vi "ge_CalibrateDynamic.vi"(5 "Chassis Name":string="cDAQ1", 7 "Selected Rows":i32[](array[numeric])=[0, 1, 2, 3], 8 "error in":errorcluster, 10 "ge_DAQManDefinitions":T1, 11 "ItemNames":string[][](array[string])=[["Mod1/ai0", "NI 9234", "", "", "F", "1000.00", "V", "2 mA", "5 V", "F", "1.000000", "1", "EU", "RMS"], ["Mod1/ai1", "NI 9234", "", "", "F", "1000.00", "V", "2 mA", "5 V", "F", "1.000000", "1", "EU", "RMS"], ["Mod1/ai2", "NI 9234", "", "", "F", "1000.00", "V", "2 mA", "5 V", "F", "1.000000", "1", "EU", "RMS"], ["Mod1/ai3", "NI 9234", "", "", "F", "1000.00", "V", "2 mA", "5 V", "F", "1.000000", "1", "EU", "RMS"]]) -> (0 "error out":errorcluster, 2 "Cell Contents":T2[](array[typedef]))   [LabVIEW 2018]
uses:
  Custom Ctls Table/ge_CellContents.ctl
  <vilib>/Utility/miscctls.llb/LVPoint32TypeDef.ctl
  Common/Controls/DAQMan Definitions.ctl
  ge_GrphTblCmnds.ctl
  Custom Ctrls/ge_MeasType.ctl
  Classes/Measurements/Class Dynamic/Dynamic.lvclass
  <vilib>/addons/_NISVFA/_Shared subVIs/Controls/svc_Window.ctl
  <vilib>/DAQmx/read.llb/DAQmx Read (Analog 1D Wfm NChan NSamp).vi
  <vilib>/addons/_NISVFA/_Spectrum Processing/SVFA Spectrum Peak Search (1 Ch).vi
  <vilib>/addons/_NISVFA/_Spectrum Processing/subVIs/svfa_Spectrum Peak Search.vi
  <vilib>/addons/_NISVFA/_Shared subVIs/Common/svc_Spectrum Units.vi
  <vilib>/addons/_NISVFA/_Spectrum Processing/subVIs/svfa_Peak Rough Search Indices.vi
  <vilib>/DAQmx/configure/timing.llb/DAQmx Timing (Sample Clock).vi
  <vilib>/DAQmx/miscellaneous.llb/DAQmx Fill In Error Info.vi
  <vilib>/addons/_NISVFA/_Baseband FFT/SVFA Power Spectrum (1 Ch).vi
  <vilib>/addons/_NISVFA/_Spectrum Processing/subVIs/svfa_Three Finger Peak Search.vi
  <vilib>/addons/_NISVFA/_Shared subVIs/Common/svc_Format Value (DBL).vi
  <vilib>/addons/_NISVFA/_Shared subVIs/Common/svc_Engineering Units to Unit Label.vi
  <vilib>/addons/_NISVFA/_Shared subVIs/Common/svc_Unit Label Lexical Class.vi
  <vilib>/addons/_NISVFA/_Shared subVIs/Common/svc_Get Weighting Enum and Labels.vi
  <vilib>/addons/_NISVFA/_Shared subVIs/Common/svc_Caller VI Returned in Error Source.vi
  <vilib>/addons/_NISVFA/_Baseband FFT/SVFA Power Spectrum (N Ch).vi
panel:
  out "Calibration Source":string
  in  "dB On (T)":bool=TRUE
  out "Calibration Freq (Hz)":dbl=2.048000000000001
  in  "Cancel":bool
  in  "Apply":bool
  in  "Accept":bool
  in  "Legend LB":i32[](listbox)=[0]
  out "Wfm Graph":cluster{"f0":dbl, "df":dbl, "magnitude":dbl[]}[](graph)=[{"f0"=0.0, "df"=2.048000000000001, "magnitude"=array[6250 elements]}, {"f0"=0.0, "df"=2.048000000000001, "magnitude"=array[6250 elements]}, {"f0"=0.0, "df"=2.048000000000001, "magnitude"=array[6250 elements]}, {"f0"=0.0, "df"=2.048000000000001, "magnitude"=array[6250 elements]}]
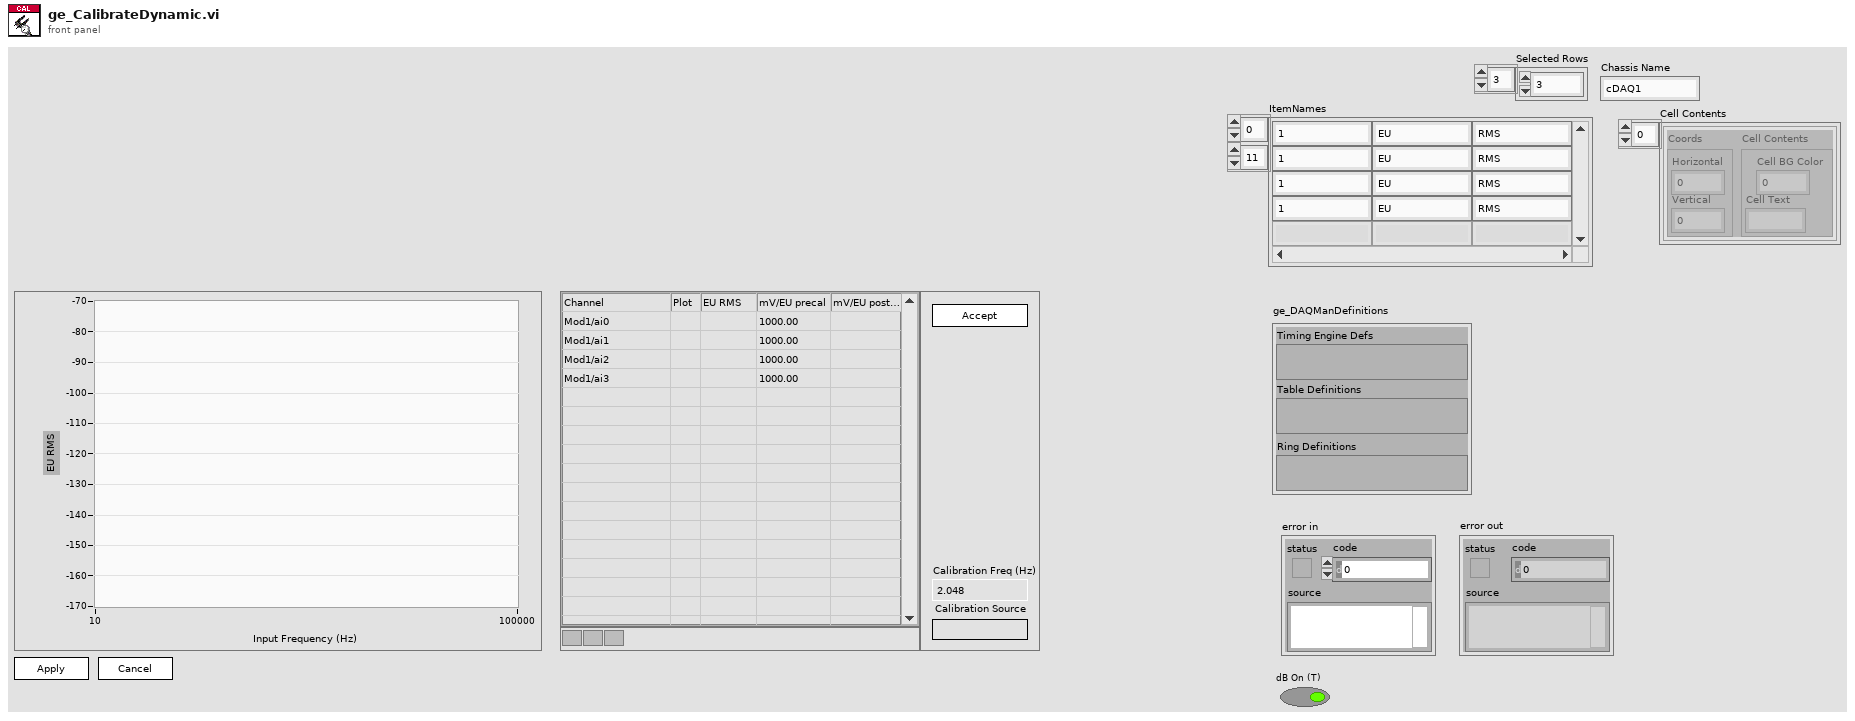
[diagram p1: front panel]
types:
  T1 = typedef "DAQMan Definitions.ctl" = cluster{"Timing Engine Defs":variant, "Table Definitions":variant, "Ring Definitions":variant}
  T2 = typedef "ge_CellContents.ctl" = cluster{"Cell Contents":cluster{"Cell Text":string, "Cell BG Color":u32}, "Coords":T3}
  T3 = typedef "LVPoint32TypeDef.ctl" = cluster{"Horizontal":i32, "Vertical":i32}
  T4 = typedef "ge_GrphTblCmnds.ctl" = enum16{"Load Refs", "Init FP", "Active Plot", "CalRef", "AcceptCal", "Scale Wfm", "Update RMS", "Update Sens", "Get Sens", "Shutdown"}
  T5 = typedef "ge_MeasType.ctl" = enum16{"Voltage", "Frequency", "Tachometer", "Dynamic", "Thermocouple", "RTD", "Strain", "Current", "Resistance"}
  T6 = cluster{"This VI":refnum<vi>, refnum<class "Dynamic.lvclass">[]}
  T7 = cluster{cluster{string, "Normal":u32}, cluster{i32, "index of element":i32}}[]
  T8 = cluster{"single/multiple":enum16{"Multiple Peaks", "Single Max Peak"}, "threshold":dbl}
  T9 = typedef "svc_Window.ctl" = u32
  T10 = typedef "svc_Spectrum Info.ctl" = cluster{"channel name":string, "description":string, "x-axis units":T11, "spectral info":cluster{"spectrum type":T12, "linear/dB":enum16{"linear", "dB"}, "window":u16, "window size":i32, "FFT size":i32}, "engineering units":T13, "custom label":string, "dB reference [EU]":dbl, "peak units":enum16{"rms", "peak", "peak-peak"}, "weighting filter":T14, "spectral density?":bool, "unit label":string, "spectrum skewed?":bool, "complimentary spectrum units":T15}
  T11 = typedef "svc_X-Axis Units.ctl" = u16
  T12 = typedef "svc_Spectrum Type.ctl" = enum16{"FFT Spectrum [complex]", "Amplitude [Magnitude]", "Power [Magnitude^2]", "Cross Spectrum [complex]", "Frequency Response [Complex]"}
  T13 = typedef "svc_Engineering Units Text Ring.ctl" = u16
  T14 = typedef "svc_Weighting Filter Text Ring.ctl" = u16
  T15 = typedef "svc_Complimentary Spectrum Units.ctl" = enum16{"none", "radians", "degrees", "cycles", "imaginary"}
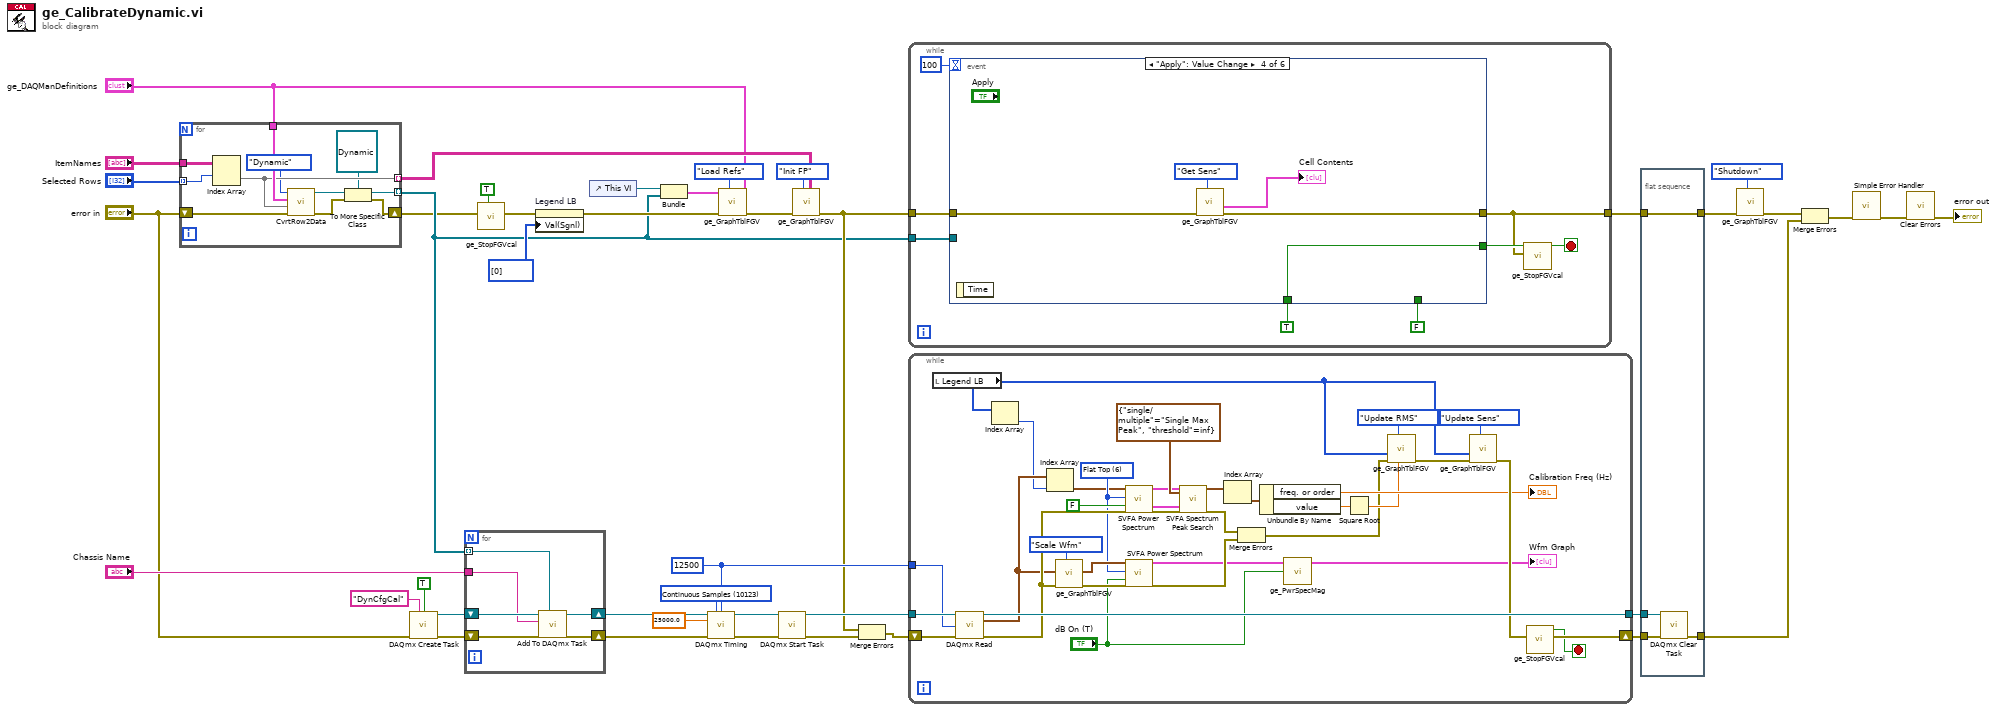
[diagram p0: block diagram]
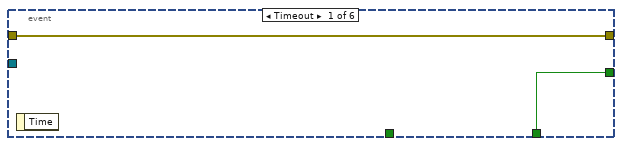
[diagram p2: hidden frame]
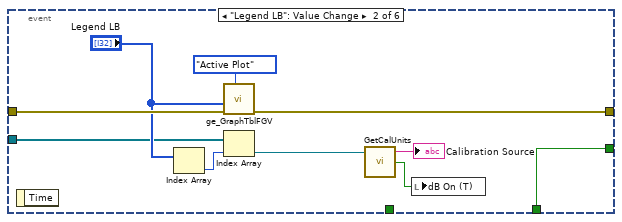
[diagram p3: hidden frame]
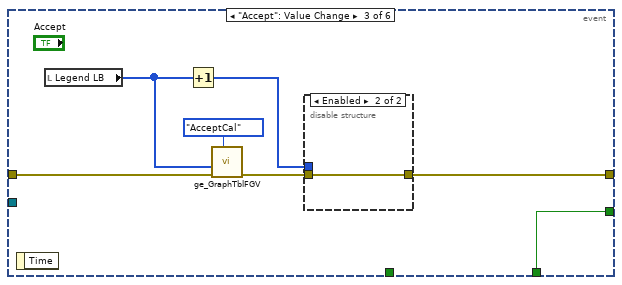
[diagram p4: hidden frame]
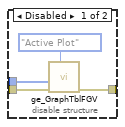
[diagram p5: hidden frame]
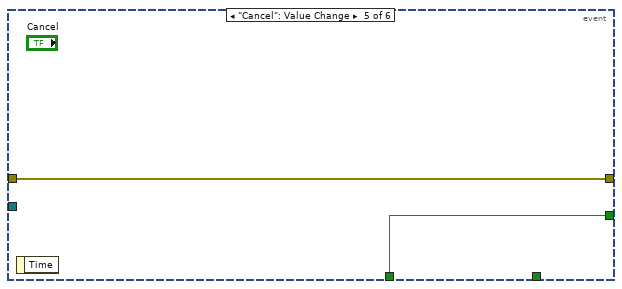
[diagram p6: hidden frame]
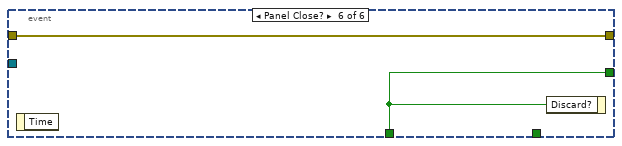
[diagram p7: hidden frame]
diagram:
  w28 = 12500 ("samples per channel")
  w35 = 10123 items=["Finite Samples"=10178, "Continuous Samples"=10123, "Hardware Timed Single Point"=12522] ("sample mode")
  n1 = for {
    tunnel: "Selected Rows" -> [w52] mode=indexing
    tunnel: "ItemNames" -> [w53]
    tunnel: [w50] -> w17 mode=indexing
    tunnel: [w47] -> w3 mode=indexing
    tunnel: "ge_DAQManDefinitions" -> [w51]
    shift-right: [w44] -> w2
    shift-left: "error in" -> [w43]
    n2 = Index Array(array=w53, index (row)=w52) -> (element=w50:string[])  [unwired: 1 in]
    n3 = call "CvrtRow2Data.vi"("error in (no error)"=w43, "Item Names"=w50, "ge_DAQManDefinitions"=w51, "MeasType"=ge_MeasType."Dynamic") -> ("error out"=w45:errorcluster, "Channel out"=w48:refnum<class "Channel.lvclass">)  [unwired: 6 in]
    n4 = To More Specific Class(target class=refnum<class "Dynamic.lvclass"> refnum ("Dynamic.lvclass"), reference=w48, error in=w45) -> (specific class reference=w47:refnum<class "Dynamic.lvclass">, error out=w44:errorcluster)
  }
  n5 = call <vilib>:"DAQmx Create Task.vi"("new task name"="DynCfgCal", "auto cleanup"=TRUE, "error in"="error in") -> ("task out"=w38:refnum<k21>, "error out"=w37:errorcluster)  [unwired: 11 in]
  n6 = for {
    shift-right: [w56] -> w33
    shift-left: w38 -> [w59]
    shift-right: [w55] -> w34
    shift-left: w37 -> [w58]
    tunnel: w3 -> [w57] mode=indexing
    tunnel: "Chassis Name" -> [w54]
    n7 = call-dynamic "Add To DAQmx Task.vi"("Dynamic in"=w57, "error in (no error)"=w58, "Chassis Name"=w54, "task in"=w59) -> ("error out"=w55:errorcluster, "task out"=w56:refnum<k21>)  [unwired: 5 in, 1 out]
  }
  n8 = call "ge_StopFGVcal.vi"("Reset (F)"=TRUE, "error in"=w2) -> ("error out"=w9:errorcluster)  [unwired: 8 in, 1 out]
  n9 = property on="Legend LB" class="MCListbox (strict)"(error in=w9, "Val(Sgnl)"=i32[] [0] ("Value (Signaling)")) -> (error out=w8:errorcluster)  [unwired: 1 in, 1 out]
  n10 = control-ref of="This VI"() -> (w12:refnum<vi>)
  n11 = Bundle("This VI"=w12, w3) -> (w11:T6)  [unwired: 1 in]
  n12 = call-poly <vilib>:"DAQmx Timing.vi"("task/channels in"=w33, "sample mode"=w35, "samples per channel"=w28, "rate"=25000.0, "error in"=w34) -> ("task out"=w31:refnum<k21>, "error out"=w30:errorcluster)  [unwired: 9 in]
  n13 = call "ge_GraphTblFGV.vi"("ge_DAQManDefinitions"="ge_DAQManDefinitions", "GrphTblCmnds"=ge_GrphTblCmnds."Load Refs", "error in"=w8, "Init Info"=w11) -> ("error out"=w21:errorcluster)  [unwired: 5 in, 2 out]
  n14 = call <vilib>:"DAQmx Start Task.vi"("task/channels in"=w31, "error in"=w30) -> ("task out"=w29:refnum<k21>, "error out"=w20:errorcluster)  [unwired: 12 in]
  n15 = call "ge_GraphTblFGV.vi"("ItemNames"=w17, "GrphTblCmnds"=ge_GrphTblCmnds."Init FP", "error in"=w21) -> ("error out"=w19:errorcluster)  [unwired: 6 in, 2 out]
  n16 = Merge Errors(w19, w20) -> (w18:errorcluster)
  n17 = while {
    tunnel: w19 -> [w62]
    tunnel: [w61] -> w16
    tunnel: w3 -> [w60]
    stop <- w64 stop-if-true
    n18 = event shown="[3] \"Apply\": Value Change" {
      selector: _ -> [_ _ _ _ _ _]
      dyn-events: _ -> [_ _ _ _ _ _]
      timeout: 100 -> [_ _ _ _ _ _]
      tunnel: TRUE ("Discard?") -> [_ _ _ w96 w98 w100]
      tunnel: FALSE ("Discard?") -> [w69 w79 w86 _ _ _]
      tunnel: [w68 w76 w82 w93 w97 w99] -> w61
      tunnel: [w69 w79 w86 w96 w98 w100] -> w65
      tunnel: w62 -> [w68 w77 w84 w94 w97 w99]
      tunnel: w60 -> [_ w74 _ _ _ _]
      event Timeout {
        n19 = event-data() -> ()  [unwired: 1 in, 1 out]
      }
      event "Legend LB": Value Change {
        n20 = event-data() -> ()  [unwired: 1 in, 1 out]
        n21 = Index Array(array="Legend LB") -> (element=w73:i32)  [unwired: 1 in]
        n22 = call "ge_GraphTblFGV.vi"("GrphTblCmnds"=ge_GrphTblCmnds."Active Plot", "error in"=w77, "Legend LB"="Legend LB") -> ("error out"=w76:errorcluster)  [unwired: 6 in, 2 out]
        n23 = Index Array(array=w74, index=w73) -> (element=w71:refnum<class "Dynamic.lvclass">)
        n24 = call "GetCalUnits.vi"("Dynamic.lvclass"=w71) -> ("Calibration Units"=→"Calibration Source":string, "dB On"=w70:bool)  [unwired: 7 in]
        n25 = local write "dB On (T)"(w70) -> ()
      }
      event "Accept": Value Change {
        n26 = event-data() -> ()  [unwired: 1 in, 1 out]
        n27 = local read "Legend LB"() -> (w81:i32[])
        n28 = Increment(x=w81) -> (x+1=w80:i32[])
        n29 = call "ge_GraphTblFGV.vi"("GrphTblCmnds"=ge_GrphTblCmnds."AcceptCal", "error in"=w84, "Legend LB"=w81) -> ("error out"=w83:errorcluster)  [unwired: 6 in, 2 out]
        n30 = disable-structure shown="Enabled" {
          disable-tunnel: w83 -> [w89 w91]
          disable-tunnel: [w88 w91] -> w82
          disable-tunnel: w80 -> [w87 _]
          frame Disabled {
            n31 = call "ge_GraphTblFGV.vi"("GrphTblCmnds"=ge_GrphTblCmnds."Active Plot", "error in"=w89, "Legend LB"=w87) -> ("error out"=w88:errorcluster)  [unwired: 6 in, 2 out]
          }
          frame Enabled {
          }
        }
      }
      event "Apply": Value Change {
        n32 = event-data() -> ()  [unwired: 1 in, 1 out]
        n33 = call "ge_GraphTblFGV.vi"("GrphTblCmnds"=ge_GrphTblCmnds."Get Sens", "error in"=w94) -> ("error out"=w93:errorcluster, "Cell Contents"=→"Cell Contents":T7)  [unwired: 7 in, 1 out]
      }
      event "Cancel": Value Change {
        n34 = event-data() -> ()  [unwired: 1 in, 1 out]
      }
      event Panel Close? {
        n35 = event-data() -> ()  [unwired: 1 in, 1 out]
        n36 = event-data("Discard?"=w100) -> ()  [unwired: 1 in, 1 out]
      }
    }
    n37 = call "ge_StopFGVcal.vi"("error in"=w61, "User stop? (F)"=w65) -> ("Stop?"=w64:bool)  [unwired: 8 in, 1 out]
  }
  n38 = while {
    shift-right: [w135] -> w27
    shift-left: w18 -> [w133]
    tunnel: w29 -> [w132]
    tunnel: w28 -> [w130]
    tunnel: [w131] -> w26
    stop <- w134 stop-if-true
    w113 = T9 6 items=["None"=0, "Hanning"=1, "Hamming"=2, "Blackman-Harris"=3, "Exact Blackman"=4, "Blackman"=5, "Flat Top"=6, "4 Term B-Harris "=7, "7 Term B-Harris"=8, "Low Sidelobe"=9, "Blackman Nuttall"=11, "Triangle"=30, "Bartlett-Hanning"=31, "Bohman"=32, "Parzen"=33, "Welch"=34, "Kaiser"=60, "Dolph-Chebyshev"=61, "Gaussian"=62] ("window")
    n39 = local read "Legend LB"() -> (w125:i32[])
    n40 = call-poly <vilib>:"DAQmx Read.vi"("task/channels in"=w132, "number of samples per channel"=w130, "error in"=w133) -> ("task out"=w131:refnum<k21>, "data"=w112:waveform(dbl)[], "error out"=w118:errorcluster)  [unwired: 10 in]
    n41 = Index Array(array=w125) -> (element=w110:i32)  [unwired: 1 in]
    n42 = Index Array(array=w112, index=w110) -> (element=w111:waveform(dbl))
    n43 = call "ge_GraphTblFGV.vi"("GrphTblCmnds"=ge_GrphTblCmnds."Scale Wfm", "error in"=w118, "Wfm In"=w112) -> ("error out"=w107:errorcluster, "Wfm Out"=w117:waveform(dbl)[])  [unwired: 6 in, 1 out]
    n44 = call-poly <vilib>:"SVFA Power Spectrum.vi"("scaled signal [EU]"=w111, "window"=w113, "dB On (T)"=FALSE, "error in (no error)"=w118) -> ("power spectrum [dB EU]"=w109:cluster{"f0":dbl, "df":dbl, "magnitude":dbl[]}, "spectrum info"=w108:T10, "error out"=w123:errorcluster)  [unwired: 10 in, 3 out]
    n45 = call-poly <vilib>:"SVFA Power Spectrum.vi"("scaled signals [EU]"=w117, "window"=w113, "dB On (T)"="dB On (T)", "error in (no error)"=w107) -> ("power spectra [dB EU]"=w103:cluster{"f0":dbl, "df":dbl, "magnitude":dbl[]}[], "error out"=w105:errorcluster)  [unwired: 10 in, 4 out]
    n46 = call-poly <vilib>:"SVFA Spectrum Peak Search.vi"("spectrum"=w109, "peak search settings"=T8 {"single/multiple"=enum."Single Max Peak", "threshold"=inf}, "spectrum info in"=w108, "error in (no error)"=w123) -> ("peaks"=w121:cluster{"freq. or order":dbl, "value":dbl}[], "error out"=w106:errorcluster)  [unwired: 11 in, 3 out]
    n47 = Index Array(array=w121) -> (element=w120:cluster{"freq. or order":dbl, "value":dbl})  [unwired: 1 in]
    n48 = Merge Errors(w106, w105) -> (w104:errorcluster)
    n49 = Unbundle By Name(w120) -> ("freq. or order"=→"Calibration Freq (Hz)":dbl, "value"=w116:dbl)
    n50 = call "ge_PwrSpecMag.vi"("dB On (T)"="dB On (T)", "power spectra [dB EU]"=w103) -> ("power spectra [dB EU]"=→"Wfm Graph":cluster{"f0":dbl, "df":dbl, "magnitude":dbl[]}[])  [unwired: 3 in]
    n51 = Square Root(x=w116) -> (sqrt(x)=w115:dbl)
    n52 = call "ge_GraphTblFGV.vi"("RMS Value"=w115, "GrphTblCmnds"=ge_GrphTblCmnds."Update RMS", "error in"=w104, "Legend LB"=w125) -> ("error out"=w127:errorcluster)  [unwired: 5 in, 2 out]
    n53 = call "ge_GraphTblFGV.vi"("GrphTblCmnds"=ge_GrphTblCmnds."Update Sens", "error in"=w127, "Legend LB"=w125) -> ("error out"=w126:errorcluster)  [unwired: 6 in, 2 out]
    n54 = call "ge_StopFGVcal.vi"("error in"=w126) -> ("error out"=w135:errorcluster, "Stop?"=w134:bool)  [unwired: 9 in]
  }
  n55 = flat-sequence {
    tunnel: w27 -> [w139]
    tunnel: w26 -> [w138]
    tunnel: [w137] -> w25
    tunnel: [w136] -> w14
    tunnel: w16 -> [w136]
    frame #0 {
      n56 = call <vilib>:"DAQmx Clear Task.vi"("task in"=w138, "error in"=w139) -> ("error out"=w137:errorcluster)  [unwired: 13 in]
    }
  }
  n57 = call "ge_GraphTblFGV.vi"("GrphTblCmnds"=ge_GrphTblCmnds."Shutdown", "error in"=w14) -> ("error out"=w13:errorcluster)  [unwired: 7 in, 2 out]
  n58 = Merge Errors(w13, w25) -> (w6:errorcluster)
  n59 = call <vilib>:"Simple Error Handler.vi"("error in (no error)"=w6) -> ("error out"=w5:errorcluster)  [unwired: 4 in, 4 out]
  n60 = call <vilib>:"Clear Errors.vi"("error in (no error)"=w5) -> ("error out"=→"error out":errorcluster)  [unwired: 5 in, 1 out]
